vi "Parse name to node.vi"(10 "error in":errorcluster, 11 "Name":string) -> (2 "error out":errorcluster, 3 "Array":string[](array[string]))   [LabVIEW 2018, in "Name and Dependency Processing.lvlib"]
uses:
  Name and Dependency Processing.lvlib
  Path and string processing/Path and String Processing.lvlib
  DGML Creation/DGML creation.lvlib
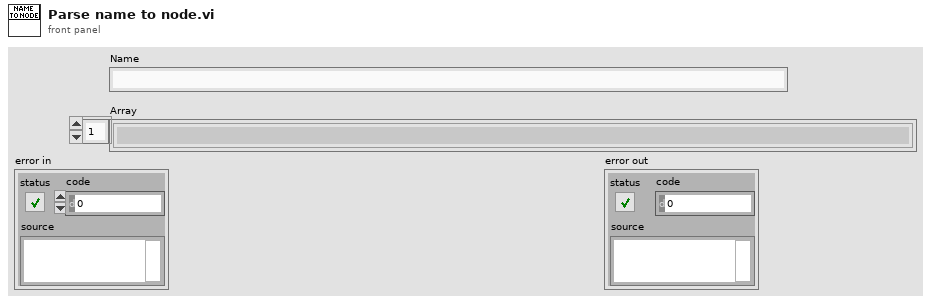
[diagram p1: front panel]
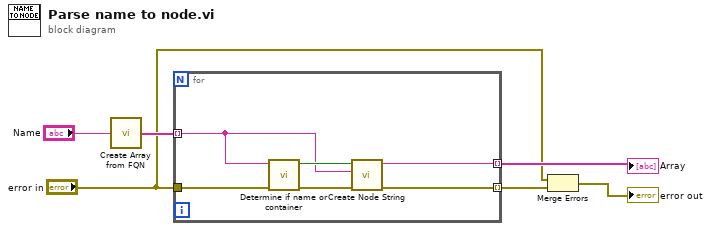
[diagram p0: block diagram]
diagram:
  n1 = call "Create Array from FQN.vi"("FQN In"="Name") -> ("Array of namespaces and name"=w5:string[])
  n2 = for {
    tunnel: w5 -> [w7] mode=indexing
    tunnel: [w12] -> w4 mode=indexing
    tunnel: [w10] -> w3 mode=indexing
    tunnel: "error in" -> [w9]
    n3 = call "Determine if name or container.vi"("error in (no error)"=w9, "Name or Namespace"=w7) -> ("error out"=w11:errorcluster, "Is Container?"=w8:bool)  [unwired: 8 in]
    n4 = call "Create Node String.vi"("error in (no error)"=w11, "token string"=w7, "Is namespace or group?"=w8) -> ("error out"=w10:errorcluster, "format string"=w12:string)  [unwired: 7 in]
  }
  "Array" <- w4
  n5 = Merge Errors("error in", w3) -> (→"error out":errorcluster)
